vi "Producer Consumer Test.vi"() -> ()   [LabVIEW 2021]
uses:
  <vilib>/Platform/TimedLoop/XDataNode/timing_clust.ctl
  <vilib>/Platform/TimedLoop/XDataNode/nitl_modes.ctl
  <vilib>/Platform/TimedLoop/XDataNode/wakeup.ctl
  <vilib>/platform/TimedLoop/XDataNode/XDataNode.xnode
  <vilib>/Platform/TimedLoop/XDataNode/XDNodeRunTimeDep.lvlib
panel:
  out "Numeric":i32
  out "x+y 2":i32
  out "Array":i32[](array[numeric])
  in  "Stop":bool
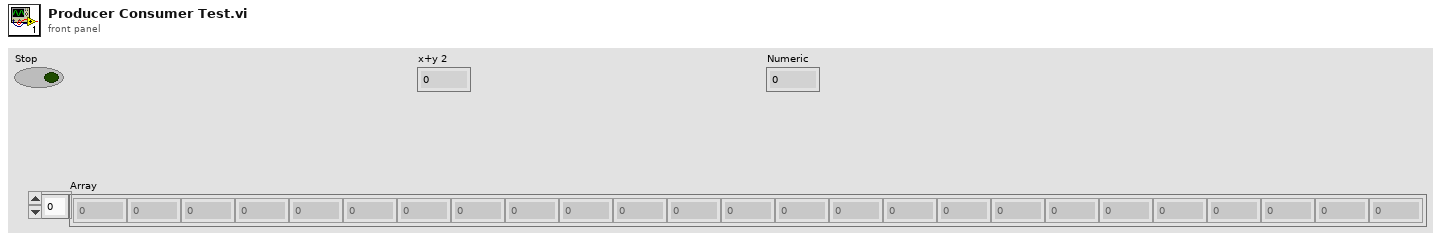
[diagram p1: front panel]
types:
  T1 = typedef "XDNodeRunTimeDep.lvlib/timing_clust.ctl" = cluster{"Expected End [f-1]":u64, "Actual End [f-1]":u64, "Finished Late? [f-1]":bool, "Expected End [i-1]":u64, "Actual End [i-1]":u64, "Finished Late? [i-1]":bool, "Expected Start [i]":u64, "Actual Start [i]":u64, "Expected Start [f]":u64, "Actual Start [f]":u64, "Source Name":string, "Structure Name":string, "Period":i64, "Deadline":i64, "Offset":i64, "Start":i64, "Priority":i32, "Timeout":i32, "Mode":T2, "Wakeup Reason":T3, "Error":errorcluster, "Source Type":string, "Secondary Source Type":string, "Global End Time":u64, "Global Start Time":u64, "Frame Duration":u64, "Iteration Duration":u64, "Assigned CPU":i32, "I/O Scan Engine Mode":u32}
  T2 = typedef "XDNodeRunTimeDep.lvlib/nitl_modes.ctl" = enum32{"No Change", "Process missed periods, maintain original phase", "Discard missed periods, maintain original phase", "Process missed periods, ignore original phase", "Discard missed periods, ignore original phase"}
  T3 = typedef "XDNodeRunTimeDep.lvlib/wakeup.ctl" = enum32{"Normal", "Aborted", "Asynchronous wakeup", "Timing source error", "Timed loop error", "Timeout"}
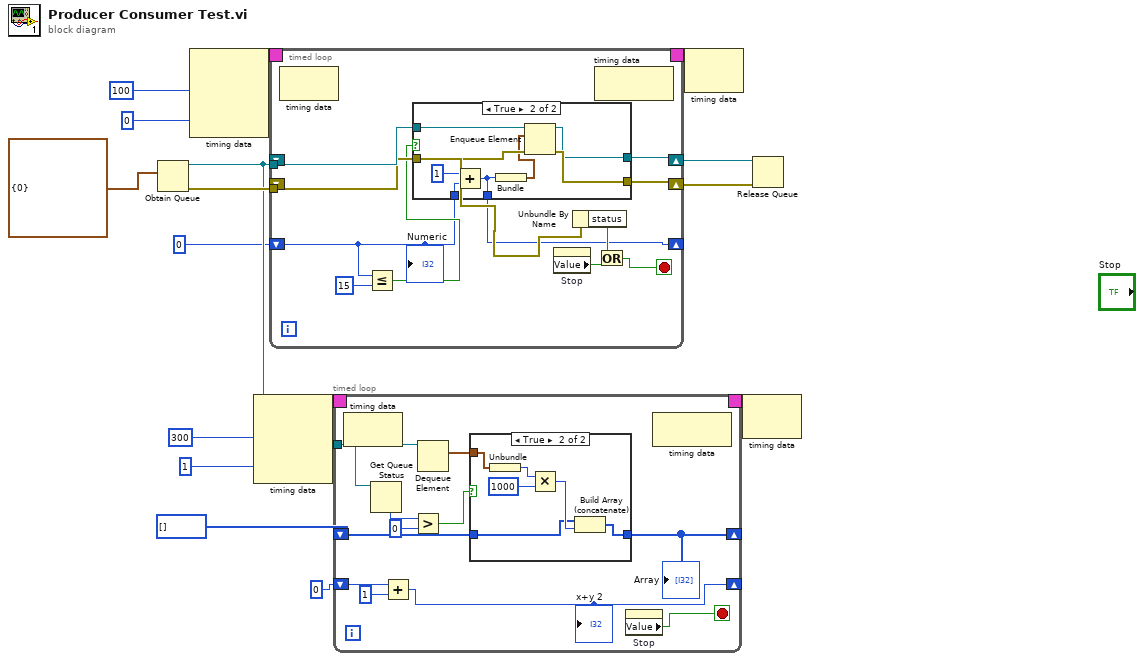
[diagram p0: block diagram]
diagram:
  n1 = Obtain Queue(element data type=cluster{i32} {0}) -> (queue out=w8:refnum<queue>, error out=w9:errorcluster)  [unwired: 4 in, 1 out]
  n2 = node-c288(i64 100 ("Period"), 0 ("Processor")) -> (w16:T1)  [unwired: 2 in]
  n3 = node-c288(i64 300 ("Period"), 1 ("Processor")) -> (w14:T1)  [unwired: 2 in]
  n4 = timed-loop {
    timing: w16 -> [_]
    timing-out: [_] -> w15
    tunnel: w8 -> [w27]
    tunnel: w9 -> [w21]
    shift-right: [w26] -> w7
    shift-left: _ -> [_]
    shift-right: [w17] -> _
    shift-left: 0 -> [w18]
    shift-right: [w24] -> w3
    shift-left: _ -> [_]
    stop <- w25 stop-if-true
    n5 = node-c288() -> ()  [unwired: 1 in, 1 out]
    n6 = Less Or Equal?(x=w18, y=15) -> (x <= y?=w19:bool)
    n7 = case shown="True" w19 {
      tunnel: w27 -> [w30 w38]
      tunnel: w21 -> [w29 w37]
      tunnel: [w29 w36] -> w26
      tunnel: [w30 w35] -> w24
      tunnel: w18 -> [w28 w32]
      tunnel: [w28 w31] -> w17
      frame False {
      }
      frame True {
        n8 = Add(x=1, y=w32) -> (x+y=w31:i32)
        n9 = Bundle(w31) -> (w33:cluster{i32})  [unwired: 1 in]
        n10 = Enqueue Element(queue=w38, element=w33, error in (no error)=w37) -> (queue out=w35:refnum<queue>, error out=w36:errorcluster)  [unwired: 1 in, 1 out]
      }
    }
    n11 = property on="Stop" class="Bool (strict)"() -> ("Value"=w22:bool)  [unwired: 2 in, 2 out]
    n12 = Unbundle By Name(w21) -> ("status"=w20:bool)
    n13 = node-c288() -> ()  [unwired: 1 in, 1 out]
    n14 = Or(x=w20, y=w22) -> (x .or. y?=w25:bool)
    "Numeric" <- w18
  }
  n15 = timed-loop {
    timing: w14 -> [_]
    timing-out: [_] -> w13
    shift-right: [w49] -> _
    shift-left: i32[] [] -> [w50]
    shift-right: [w46] -> _
    shift-left: 0 -> [w48]
    tunnel: w8 -> [w43]
    stop <- w41 stop-if-true
    n16 = node-c288() -> ()  [unwired: 1 in, 1 out]
    n17 = Get Queue Status(queue=w43) -> (# elements in queue=w44:i32)  [unwired: 2 in, 7 out]
    n18 = Add(x=w48, y=1) -> (x+y=w46:i32)
    "x+y 2" <- w46
    n19 = Greater?(x=w44, y=0) -> (0:w42:bool)
    n20 = Dequeue Element(queue=w43) -> (element=w51:cluster{i32})  [unwired: 2 in, 3 out]
    n21 = case shown="True" w42 {
      tunnel: w51 -> [_ w58]
      tunnel: w50 -> [w52 w54]
      tunnel: [w52 w53] -> w49
      frame False {
      }
      frame True {
        n22 = Unbundle(w58) -> (w57:i32)
        n23 = Multiply(x=w57, y=1000) -> (x*y=w55:i32)
        n24 = Build Array (concatenate)(w54, w55) -> (w53:i32[])
      }
    }
    "Array" <- w49
    n25 = property on="Stop" class="Bool (strict)"() -> ("Value"=w41:bool)  [unwired: 2 in, 2 out]
    n26 = node-c288() -> ()  [unwired: 1 in, 1 out]
  }
  n27 = node-c288(w15) -> ()  [unwired: 1 out]
  n28 = node-c288(w13) -> ()  [unwired: 1 out]
  n29 = Release Queue(queue=w3, error in (no error)=w7) -> ()  [unwired: 1 in, 3 out]
